vi "shag_start — 10.vi"() -> ()   [LabVIEW 2016]
uses:
  <vilib>/Instr/_visa.llb/VISA Configure Serial Port (Instr).vi
panel:
  out "положение в мин 4":i32
  out "text4":string
  out "4":i32
  out "3":i32
  out "положение в мин 3":i32
  out "text3":string
  out "text":string
  out "2":i32
  out "1":i32
  out "text2":string
  out "положение в мин 2":i32
  out "положение в мин 1":i32
  in  "all":T1(tab)
  out "положение шд 2":i32(knob) scale=-10.0..190.0
  out "текущее положение 2":string
  out "положение в минутах 2":string
  in  "Минуты 2":i32 min=-600 max=11400
  in  "Stop двигатель 2":bool
  in  "Вращение по градусам +  2":bool
  in  "Вращение по градусам -  2":bool
  in  "Вернуться в нулевое положение 2":bool
  in  "Задать текущее положение нулевым 2":bool
  in  "Установка минут 2":bool
  in  "Блокировать трубку №2":bool
  out "положение шд":i32(knob) scale=-10.0..190.0
  out "текущее положение":string
  out "положение в минутах 1":string
  in  "Минуты":i32 min=-600 max=11400
  in  "Stop двигатель":bool
  in  "Вращение по градусам +":bool
  in  "Вращение по градусам -":bool
  in  "Вернуться в нулевое положение":bool
  in  "Задать текущее положение нулевым":bool
  in  "Установка минут":bool
  in  "Блокировать зеркало №1":bool
  in  "stop":bool
  out "положение шд 3":i32(knob) scale=-10.0..190.0
  out "текущее положение 3":string
  out "положение в минутах 3":string
  in  "Минуты 3":i32 min=-600 max=11400
  in  "Stop двигатель 3":bool
  in  "Вращение по градусам +  3":bool
  in  "Вращение по градусам -  3":bool
  in  "Вернуться в нулевое положение 3":bool
  in  "Задать текущее положение нулевым 3":bool
  in  "Установка минут 3":bool
  in  "Блокировать стол №3":bool caption="Блокировать трубку №2"
  out "положение шд 4":i32(knob) scale=-10.0..190.0
  out "текущее положение 4":string
  out "положение в минутах 4":string
  in  "Минуты 4":i32 min=-600 max=11400
  in  "Stop двигатель 4":bool
  in  "Вращение по градусам +  4":bool
  in  "Вращение по градусам -  4":bool
  in  "Вернуться в нулевое положение 4":bool
  in  "Задать текущее положение нулевым 4":bool
  in  "Установка минут 4":bool
  in  "Блокировать стол №3 2":bool caption="Блокировать трубку №2"
  in  "Выберете COM порт":refnum<visa-resource-name>="COM1"
  in  "Скорость обмена данными":u32(ring)=19200 items=["9600"=9600, "19200"=19200, "38400"=38400, "57600"=57600]
  in  "Число бит на символ":u16=8 min=5 max=8 step=1
  in  "Контроль чётности":enum16{"None", "Odd", "Even", "Mark", "Space"}(ring)
  in  "Стоповый бит":u16(ring)=10 items=["1.0"=10, "1.5"=15, "2.0"=20]
  in  "Контроль переполнения":u16(ring) items=["None"=0, "XON/XOFF"=1, "RTS/CTS"=2, "DTR/DSR"=4]
  # "1 - адресс 1 двигателя\n2 - адресс 2 двигателя\n$0MV\\01+   - запуск всех двигателей в положительном направлении \n$0MS\\00   - остановка всех двигателей\n$0MJ\\04+\\00\\00\\01   - 1 шаг всех двигателей\n$0SS\\01\\10   - скорость 10 для всех двигателей"
  # "Ренгеновская трубка №2"
  # "Положение:"
  # "Зеркало №1"
  # "Положение:"
  # "Поворотный стол №3"
  # "Положение:"
  # "Счётчик №4"
  # "Положение:"
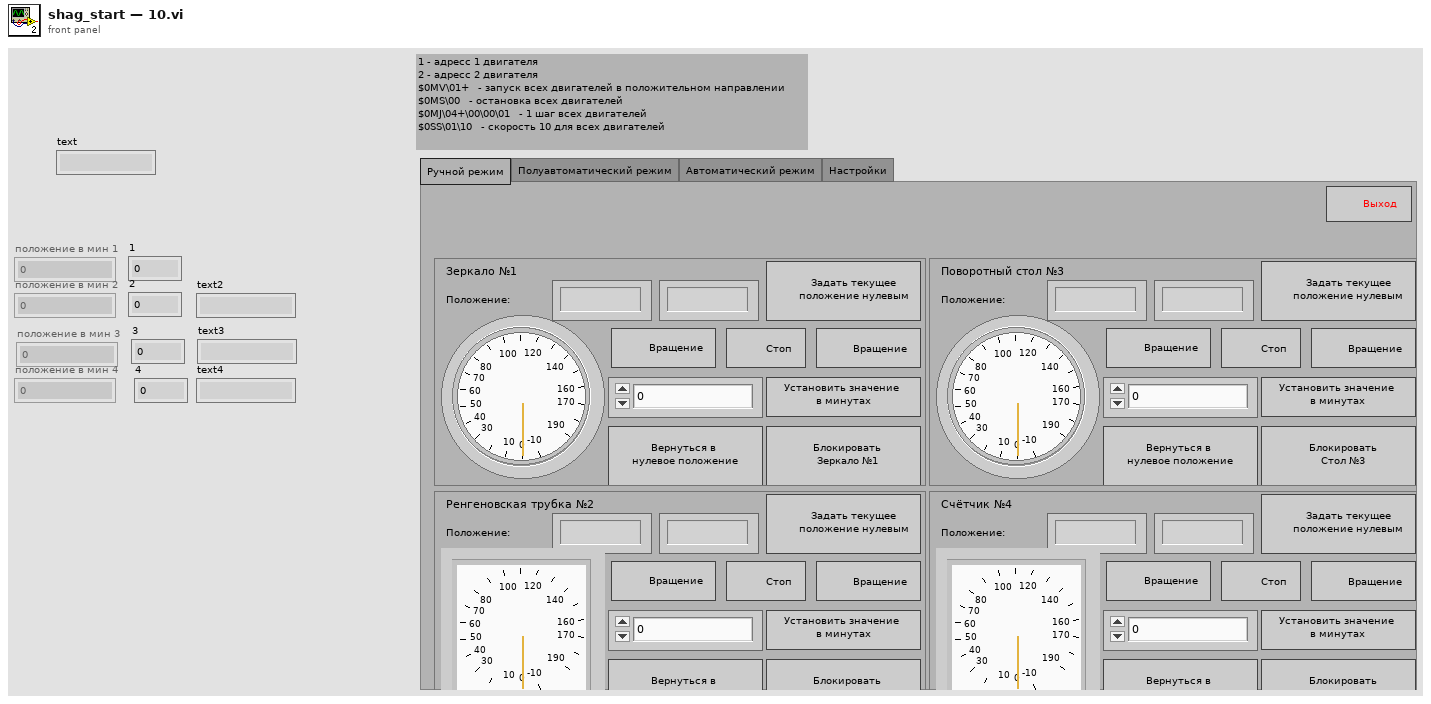
[diagram p1: front panel]
types:
  T1 = enum32{"Ручной режим", "Полуавтоматический режим", "Автоматический режим", "Настройки"}
  T2 = enum16{"open", "replace", "create", "open or create", "replace or create", "replace or create with confirmation"}
  T3 = enum8{"Enabled", "Disabled", "Disabled and Grayed Out"}
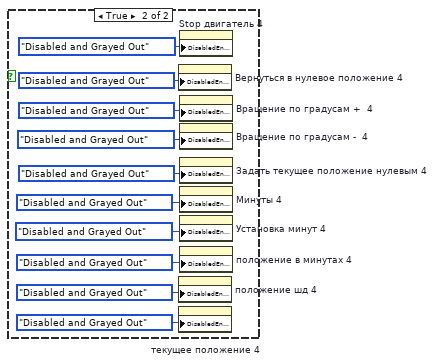
[diagram p2: hidden frame]
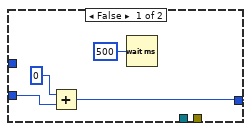
[diagram p4: hidden frame]
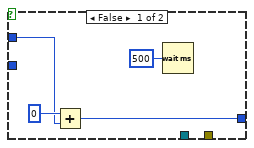
[diagram p5: hidden frame]
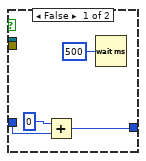
[diagram p7: hidden frame]
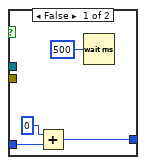
[diagram p8: hidden frame]
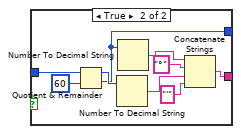
[diagram p9: hidden frame]
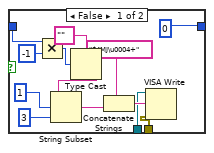
[diagram p11: hidden frame]
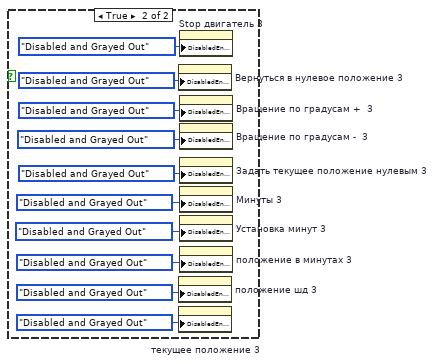
[diagram p13: hidden frame]
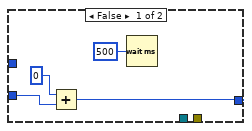
[diagram p15: hidden frame]
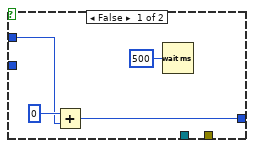
[diagram p16: hidden frame]
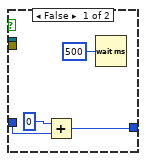
[diagram p18: hidden frame]
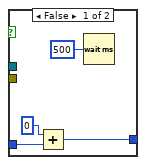
[diagram p19: hidden frame]
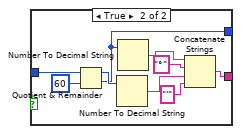
[diagram p20: hidden frame]
diagram:
  n1 = call-poly "VISA Configure Serial Port"("VISA resource name"="Выберете COM порт", "baud rate (9600)"="Скорость обмена данными", "data bits (8)"="Число бит на символ", "parity (0:none)"="Контроль чётности", "stop bits (10: 1 bit)"="Стоповый бит", "flow control (0:none)"="Контроль переполнения") -> ("VISA resource name out"=w32:refnum<visa-resource-name>, "error out"=w31:errorcluster)  [unwired: 8 in]
  n2 = Boolean To (0,1)(Boolean=FALSE ("DTR Write")) -> (0, 1=w33:i16)
  n3 = Boolean To (0,1)(Boolean=FALSE ("DTR Write")) -> (0, 1=w34:i16)
  n4 = property class="Instr"(reference=w32, error in=w31, "Serial Settings:Modem Line Settings:Line DTR State"=w33, "Serial Settings:Modem Line Settings:Line RTS State"=w34) -> (reference out=w30:refnum<visa-resource-name>, error out=w29:errorcluster)
  n5 = flat-sequence {
    tunnel: w30 -> [w63]
    tunnel: w29 -> [w62]
    tunnel: [w63] -> w28
    tunnel: [w62] -> w27
    tunnel: [w58] -> w18
    tunnel: [w66] -> w17
    tunnel: w28 -> [w66]
    tunnel: w27 -> [w65]
    tunnel: [w65] -> w15
    tunnel: [w66] -> w13
    tunnel: [w65] -> w11
    tunnel: w18 -> [w67]
    tunnel: [w65] -> w6
    tunnel: [w66] -> w5
    tunnel: [w66] -> w3
    tunnel: [w65] -> w1
    tunnel: w17 -> [w80]
    tunnel: [w80] -> w16
    tunnel: w15 -> [w79]
    tunnel: [w79] -> w14
    tunnel: w13 -> [w72]
    tunnel: [w72] -> w12
    tunnel: w11 -> [w74]
    tunnel: [w74] -> w10
    tunnel: [w75] -> w9
    tunnel: [w73] -> w8
    tunnel: [w71] -> w7
    tunnel: w6 -> [w73]
    tunnel: w5 -> [w71]
    tunnel: [w70] -> w4
    tunnel: w3 -> [w70]
    tunnel: [w69] -> w2
    tunnel: w1 -> [w69]
    tunnel: w16 -> [w90]
    tunnel: w14 -> [w89]
    tunnel: w12 -> [w85]
    tunnel: w10 -> [w88]
    tunnel: w9 -> [w87]
    tunnel: w8 -> [w84]
    tunnel: w7 -> [w83]
    tunnel: w4 -> [w82]
    tunnel: w2 -> [w81]
    frame #0 {
      n6 = VISA Write(VISA resource name=w63, write buffer="$0SS\u0001\u0010", error in (no error)=w62) -> ()  [unwired: 3 out]
      n7 = Open/Create/Replace File(file path (use dialog)=path "C:/Users/User/Desktop/shagovi_dvigatel/test_text_file", operation (0:open)=T2."open", access (0:read/write)=enum16{"read/write", "read-only", "write-only"}."read-only") -> (refnum out=w57:refnum<file>)  [unwired: 3 in, 2 out]
      n8 = Read from Text File(file (use dialog)=w57) -> (refnum out=w58:refnum<file>, text=w44:string)  [unwired: 3 in, 2 out]
      "text" <- w44
      n9 = Spreadsheet String To Array(delimiter (Tab)=" ", format string="%5f", spreadsheet string=w44) -> (array=w54:dbl[][])  [unwired: 1 in]
      n10 = Index Array(array=w54, index (row)=0 ("index")) -> (element=w52:dbl[])  [unwired: 1 in]
      n11 = Decimate 1D Array(w52) -> (w49:dbl[], w40:dbl[], w39:dbl[], w35:dbl[])
      n12 = Index Array(array=w35, index=0) -> (element=w37:dbl)
      n13 = Index Array(array=w39, index=0) -> (element=w42:dbl)
      n14 = Index Array(array=w40, index=0) -> (element=w48:dbl)
      n15 = To Long Integer(number=w37) -> (32bit integer=→"4":i32)
      n16 = To Long Integer(number=w42) -> (32bit integer=→"3":i32)
      n17 = Index Array(array=w49, index=0) -> (element=w47:dbl)
      n18 = To Long Integer(number=w48) -> (32bit integer=→"2":i32)
      n19 = To Long Integer(number=w47) -> (32bit integer=→"1":i32)
    }
    frame #1 {
      n20 = Close File(refnum=w67) -> ()  [unwired: 1 in, 2 out]
      n21 = Wait (ms)(milliseconds to wait=u32 500) -> ()  [unwired: 1 out]
    }
    frame #2 {
      n22 = Open/Create/Replace File(file path (use dialog)=path "C:/Users/User/Desktop/shagovi_dvigatel/test_text_file", operation (0:open)=T2."replace or create", access (0:read/write)=enum16{"read/write", "read-only", "write-only"}."write-only") -> (refnum out=w75:refnum<file>)  [unwired: 3 in, 2 out]
    }
    frame #3 {
      n23 = while {
        tunnel: w90 -> [w197]
        tunnel: w89 -> [w196]
        shift-right: [w192] -> _
        shift-left: _ -> [w201]
        shift-right: [w193] -> _
        shift-left: _ -> [w200]
        shift-right: [w194] -> _
        shift-left: _ -> [w199]
        shift-right: [w195] -> _
        shift-left: _ -> [w198]
        tunnel: w88 -> [w166]
        shift-right: [w188] -> w86
        shift-left: w87 -> [w189]
        tunnel: w85 -> [w165]
        shift-right: [w161] -> _
        shift-left: _ -> [w162]
        shift-right: [w159] -> _
        shift-left: _ -> [w160]
        shift-right: [w157] -> _
        shift-left: _ -> [w158]
        shift-right: [w155] -> _
        shift-left: _ -> [w156]
        tunnel: w84 -> [w133]
        tunnel: w83 -> [w132]
        shift-right: [w129] -> _
        shift-left: _ -> [w130]
        shift-right: [w127] -> _
        shift-left: _ -> [w128]
        shift-right: [w125] -> _
        shift-left: _ -> [w126]
        shift-right: [w123] -> _
        shift-left: _ -> [w124]
        tunnel: w82 -> [w101]
        tunnel: w81 -> [w100]
        shift-right: [w97] -> _
        shift-left: _ -> [w98]
        shift-right: [w95] -> _
        shift-left: _ -> [w96]
        shift-right: [w93] -> _
        shift-left: _ -> [w94]
        shift-right: [w91] -> _
        shift-left: _ -> [w92]
        stop <- "stop" stop-if-true
        # "Управление вращением"
        # "Управление вращением"
        n24 = flat-sequence {
          tunnel: w133 -> [w522]
          tunnel: w132 -> [w523]
          tunnel: [w523] -> w154
          tunnel: [w522] -> w153
          tunnel: ["Вращение по градусам +  3"] -> w152
          tunnel: ["Вращение по градусам -  3"] -> w151
          tunnel: ["Вернуться в нулевое положение 3"] -> w150
          tunnel: ["Задать текущее положение нулевым 3"] -> w149
          tunnel: ["Установка минут 3"] -> w148
          tunnel: w154 -> [w547]
          tunnel: w153 -> [w531]
          tunnel: [w570] -> w147
          tunnel: w130 -> [w567]
          tunnel: w128 -> [w569]
          tunnel: [w568] -> w146
          tunnel: w126 -> [w566]
          tunnel: w124 -> [w565]
          tunnel: w152 -> [w551]
          tunnel: w151 -> [w550]
          tunnel: [w564] -> w145
          tunnel: [w563] -> w144
          tunnel: [w548] -> w143
          tunnel: w150 -> [w548]
          tunnel: [w531] -> w142
          tunnel: [w547] -> w141
          tunnel: [w546] -> w140
          tunnel: w149 -> [w546]
          tunnel: w148 -> [w540]
          tunnel: [w529] -> w139
          tunnel: w147 -> [w654]
          tunnel: w146 -> [w655]
          tunnel: [w672] -> w138
          tunnel: [w670] -> w137
          tunnel: w145 -> [w656]
          tunnel: w144 -> [w657]
          tunnel: [w661] -> w136
          tunnel: [w668] -> w135
          tunnel: w143 -> [w664]
          tunnel: w142 -> [w660]
          tunnel: w141 -> [w659]
          tunnel: w140 -> [w658]
          tunnel: [w658] -> w134
          tunnel: w139 -> [w644]
          tunnel: [w752] -> w129
          tunnel: [w749] -> w127
          tunnel: w138 -> [w751]
          tunnel: w137 -> [w750]
          tunnel: [w748] -> w125
          tunnel: [w747] -> w123
          tunnel: w136 -> [w746]
          tunnel: w135 -> [w745]
          tunnel: w134 -> [w744]
          frame #0 {
            n25 = Wait Until Next ms Multiple(millisecond multiple=u32 300) -> ()  [unwired: 1 out]
          }
          frame #1 {
            # "Остановка двигателя"
            n26 = Greater?(x="Минуты 3", y=0) -> (0:w538:bool)
            n27 = case shown="True" "Stop двигатель 3" {
              tunnel: w547 -> [_ w618]
              tunnel: w531 -> [_ w617]
              frame False {
              }
              frame True {
                n28 = Wait (ms)(milliseconds to wait=u32 500) -> ()  [unwired: 1 out]
                n29 = VISA Write(VISA resource name=w618, write buffer="$3MS\u0001", error in (no error)=w617) -> ()  [unwired: 3 out]
              }
            }
            n30 = Not Equal?(x="Минуты 3", y=0) -> (x != y?=w537:bool)
            n31 = local read "положение в мин 3"() -> (w530:i32)
            n32 = Add(x="Минуты 3", y=w530) -> (x+y=w561:i32)
            n33 = Add(x="Минуты 3", y=w530) -> (x+y=w533:i32)
            n34 = Not Equal?(x="Минуты 3", y=0) -> (x != y?=w535:bool)
            n35 = Add(x=w530, y=60) -> (x+y=w556:i32)
            n36 = Subtract(x=w530, y=60) -> (x-y=w543:i32)
            n37 = Not(x=w538) -> (.not. x?=w539:bool)
            n38 = Greater Or Equal?(x=w533, y=-600) -> (x >= y?=w534:bool)
            n39 = Less Or Equal?(x=w561, y=11400) -> (x <= y?=w536:bool)
            n40 = Less Or Equal?(x=w556, y=11390) -> (x <= y?=w553:bool)
            n41 = Greater Or Equal?(x=w543, y=-590) -> (x >= y?=w544:bool)
            n42 = Compound Arithmetic op=AND(w539, w535, w534) -> (w557:bool)
            n43 = And(x=w551, y=w553) -> (x .and. y?=w552:bool)
            n44 = And(x=w550, y=w544) -> (x .and. y?=w549:bool)
            n45 = Compound Arithmetic op=AND(w538, w537, w536) -> (w559:bool)
            n46 = case shown="True" w540 {
              tunnel: [w573 w582] -> w570
              tunnel: w569 -> [w572 w581]
              tunnel: [w572 w580] -> w568
              tunnel: w567 -> [w573 w579]
              tunnel: w559 -> [_ w578]
              tunnel: w557 -> [_ w577]
              tunnel: w531 -> [_ w576]
              tunnel: w547 -> [_ w575]
              tunnel: "Минуты 3" -> [_ w574]
              frame False {
              }
              frame True {
                n47 = case shown="True" w578 {
                  tunnel: [w603 w609] -> w582
                  tunnel: w579 -> [w602 w608]
                  tunnel: w576 -> [_ w607]
                  tunnel: w575 -> [_ w606]
                  tunnel: w574 -> [_ w605]
                  frame False {
                    n48 = Add(x=0, y=w602) -> (x+y=w603:i32)
                    n49 = Wait (ms)(milliseconds to wait=u32 500) -> ()  [unwired: 1 out]
                  }
                  frame True {
                    n50 = Type Cast(type="", x=w605) -> (*(type *) &x=w612:string)
                    n51 = Add(x=w605, y=w608) -> (x+y=w609:i32)
                    n52 = String Subset(string=w612, offset (0)=1, length (rest)=3 ("length (rest)")) -> (substring=w611:string)
                    n53 = Concatenate Strings("$3MJ\u0004+" ("write buffer"), w611) -> (w615:string)
                    n54 = VISA Write(VISA resource name=w606, write buffer=w615, error in (no error)=w607) -> ()  [unwired: 3 out]
                  }
                }
                n55 = case shown="True" w577 {
                  tunnel: [w585 w591] -> w580
                  tunnel: w581 -> [w584 w590]
                  tunnel: w575 -> [_ w593]
                  tunnel: w576 -> [_ w592]
                  tunnel: w574 -> [_ w587]
                  frame False {
                    n56 = Add(x=0, y=w584) -> (x+y=w585:i32)
                    n57 = Wait (ms)(milliseconds to wait=u32 500) -> ()  [unwired: 1 out]
                  }
                  frame True {
                    n58 = Multiply(x=w587, y=-1) -> (x*y=w589:i32)
                    n59 = Type Cast(type="", x=w589) -> (*(type *) &x=w596:string)
                    n60 = Add(x=w590, y=w587) -> (x+y=w591:i32)
                    n61 = String Subset(string=w596, offset (0)=1, length (rest)=3 ("length (rest)")) -> (substring=w595:string)
                    n62 = Concatenate Strings("$3MJ\u0004-" ("write buffer"), w595) -> (w599:string)
                    n63 = VISA Write(VISA resource name=w593, write buffer=w599, error in (no error)=w592) -> ()  [unwired: 3 out]
                  }
                }
              }
            }
            n64 = case shown="True" w552 {
              tunnel: [w633 w640] -> w564
              tunnel: w566 -> [w632 w635]
              tunnel: w547 -> [_ w636]
              tunnel: w531 -> [_ w637]
              frame False {
                n65 = Add(x=0, y=w632) -> (x+y=w633:i32)
                n66 = Wait (ms)(milliseconds to wait=u32 500) -> ()  [unwired: 1 out]
              }
              frame True {
                n67 = VISA Write(VISA resource name=w636, write buffer="$3MJ\u0004+\u0000\u0000<", error in (no error)=w637) -> ()  [unwired: 3 out]
                n68 = Add(x=60, y=w635) -> (x+y=w640:i32)
              }
            }
            n69 = case shown="True" w549 {
              tunnel: [w623 w626] -> w563
              tunnel: w565 -> [w622 w625]
              tunnel: w547 -> [_ w629]
              tunnel: w531 -> [_ w628]
              frame False {
                n70 = Add(x=0, y=w622) -> (x+y=w623:i32)
                n71 = Wait (ms)(milliseconds to wait=u32 500) -> ()  [unwired: 1 out]
              }
              frame True {
                n72 = Subtract(x=w625, y=60 ("x")) -> (x-y=w626:i32)
                n73 = VISA Write(VISA resource name=w629, write buffer="$3MJ\u0004-\u0000\u0000<", error in (no error)=w628) -> ()  [unwired: 3 out]
              }
            }
            n74 = for {
              N: 1 -> [_]
              tunnel: [w571] -> w527 mode=indexing
              n75 = local read "3"() -> (w571:i32)
            }
            n76 = Index Array(array=w527, index=0) -> (element=w529:i32)
          }
          frame #2 {
            # "Нулевое положение"
            n77 = Add(x=w656, y=w657) -> (x+y=w665:i32)
            n78 = Add(x=w654, y=w655) -> (x+y=w669:i32)
            n79 = Add(x=w669, y=w665) -> (x+y=w650:i32)
            n80 = Add(x=w650, y=w644) -> (x+y=w649:i32)
            n81 = Not Equal?(x=w649, y=0 ("x")) -> (x != y?=w662:bool)
            n82 = And(x=w662, y=w664) -> (x .and. y?=w671:bool)
            n83 = case shown="True" w671 {
              tunnel: [w696 w719] -> w646
              tunnel: w654 -> [w700 w716]
              tunnel: [w700 w715] -> w672
              tunnel: [w699 w714] -> w670
              tunnel: w649 -> [w696 w708]
              tunnel: [w697 w710] -> w668
              tunnel: [w698 w707] -> w661
              tunnel: w655 -> [w699 w706]
              tunnel: w660 -> [_ w705]
              tunnel: w659 -> [_ w704]
              tunnel: w656 -> [w698 w703]
              tunnel: w657 -> [w697 w702]
              frame False {
              }
              frame True {
                n84 = Greater?(x=w708, y=0) -> (0:w709:bool)
                n85 = Multiply(x=w702, y=0) -> (x*y=w710:i32)
                n86 = Multiply(x=w706, y=0) -> (x*y=w714:i32)
                n87 = case shown="False" w709 {
                  tunnel: w708 -> [w724 w737]
                  tunnel: [0 0] -> w719
                  tunnel: w704 -> [w721 w734]
                  tunnel: w705 -> [w720 w733]
                  frame False {
                    n88 = Multiply(x=w724, y=-1) -> (x*y=w722:i32)
                    n89 = Type Cast(type="", x=w722) -> (*(type *) &x=w728:string)
                    n90 = String Subset(string=w728, offset (0)=1, length (rest)=3 ("length (rest)")) -> (substring=w727:string)
                    n91 = Concatenate Strings("$3MJ\u0004+" ("write buffer"), w727) -> (w731:string)
                    n92 = VISA Write(VISA resource name=w721, write buffer=w731, error in (no error)=w720) -> ()  [unwired: 3 out]
                  }
                  frame True {
                    n93 = Type Cast(type="", x=w737) -> (*(type *) &x=w740:string)
                    n94 = String Subset(string=w740, offset (0)=1, length (rest)=3 ("length (rest)")) -> (substring=w739:string)
                    n95 = Concatenate Strings("$3MJ\u0004-" ("write buffer"), w739) -> (w735:string)
                    n96 = VISA Write(VISA resource name=w734, write buffer=w735, error in (no error)=w733) -> ()  [unwired: 3 out]
                  }
                }
                n97 = local write "3"(0 ("3")) -> ()
                n98 = Multiply(x=w703, y=0) -> (x*y=w707:i32)
                n99 = Multiply(x=w716, y=0) -> (x*y=w715:i32)
              }
            }
            "положение в мин 3" <- w646
            n100 = Greater?(x=w646, y=0) -> (0:w667:bool)
            n101 = Number To Decimal String(number=w646, width (-)=i16 1) -> (decimal integer string=w652:string)
            n102 = case shown="False" w667 {
              tunnel: w646 -> [w679 w695]
              tunnel: [w683 w689] -> w643
              tunnel: [w673 w687] -> w641
              frame False {
                n103 = Multiply(x=-1, y=w679) -> (x*y=w678:i32)
                n104 = Quotient & Remainder(x=w678, y=60) -> (x-y*floor(x/y)=w682:i32, floor(x/y)=w674:i32)
                n105 = Multiply(x=-1, y=w674) -> (x*y=w673:i32)
                n106 = Number To Decimal String(number=w674) -> (decimal integer string=w680:string)  [unwired: 1 in]
                n107 = Number To Decimal String(number=w682) -> (decimal integer string=w681:string)  [unwired: 1 in]
                n108 = Concatenate Strings("-" ("string"), w680, "°" ("string"), w681, "'" ("string")) -> (w683:string)
              }
              frame True {
                n109 = Quotient & Remainder(x=w695, y=60) -> (x-y*floor(x/y)=w688:i32, floor(x/y)=w687:i32)
                n110 = Number To Decimal String(number=w688) -> (decimal integer string=w690:string)  [unwired: 1 in]
                n111 = Number To Decimal String(number=w687) -> (decimal integer string=w691:string)  [unwired: 1 in]
                n112 = Concatenate Strings(w691, "°" ("string"), w690, "'" ("string")) -> (w689:string)
              }
            }
            "текущее положение 3" <- w643
            "положение шд 3" <- w641
            n113 = Concatenate Strings(w652, "'" ("string")) -> (→"положение в минутах 3":string)
            n114 = Format Into String(w646) -> (resulting string=w647:string)  [unwired: 3 in, 1 out]
            n115 = call <vilib>:"Space Constant.vi"() -> ("String"=w645:string)
            n116 = Concatenate Strings(w645, w647) -> (→"text3":string)
          }
          frame #3 {
            # "Задача нуля"
            n117 = case shown="True" w744 {
              tunnel: [w756 w768] -> w752
              tunnel: w751 -> [w756 w769]
              tunnel: w750 -> [w755 w765]
              tunnel: [w755 w764] -> w749
              tunnel: [w754 w761] -> w748
              tunnel: [w753 w760] -> w747
              tunnel: w746 -> [w754 w759]
              tunnel: w745 -> [w753 w758]
              frame False {
              }
              frame True {
                n118 = Multiply(x=w765, y=0) -> (x*y=w764:i32)
                n119 = Multiply(x=w769, y=0) -> (x*y=w768:i32)
                n120 = Multiply(x=w758, y=0) -> (x*y=w760:i32)
                n121 = Multiply(x=w759, y=0) -> (x*y=w761:i32)
                n122 = local write "3"(0 ("3")) -> ()
              }
            }
          }
        }
        n123 = flat-sequence {
          tunnel: w196 -> [w1070]
          tunnel: w197 -> [w1071]
          tunnel: [w1071] -> w221
          tunnel: [w1070] -> w220
          tunnel: ["Вращение по градусам +"] -> w219
          tunnel: ["Вращение по градусам -"] -> w218
          tunnel: ["Вернуться в нулевое положение"] -> w217
          tunnel: ["Задать текущее положение нулевым"] -> w216
          tunnel: ["Установка минут"] -> w215
          tunnel: w221 -> [w1095]
          tunnel: w220 -> [w1077]
          tunnel: [w1118] -> w214
          tunnel: w201 -> [w1115]
          tunnel: w200 -> [w1117]
          tunnel: [w1116] -> w213
          tunnel: w199 -> [w1114]
          tunnel: w198 -> [w1113]
          tunnel: w219 -> [w1099]
          tunnel: w218 -> [w1098]
          tunnel: [w1112] -> w212
          tunnel: [w1111] -> w211
          tunnel: [w1096] -> w210
          tunnel: w217 -> [w1096]
          tunnel: [w1077] -> w209
          tunnel: [w1095] -> w208
          tunnel: [w1094] -> w207
          tunnel: w216 -> [w1094]
          tunnel: w215 -> [w1088]
          tunnel: [w1075] -> w190
          tunnel: w214 -> [w1200]
          tunnel: w213 -> [w1201]
          tunnel: [w1220] -> w206
          tunnel: [w1218] -> w205
          tunnel: w212 -> [w1202]
          tunnel: w211 -> [w1203]
          tunnel: [w1209] -> w204
          tunnel: [w1216] -> w203
          tunnel: w210 -> [w1212]
          tunnel: w209 -> [w1208]
          tunnel: w208 -> [w1207]
          tunnel: w207 -> [w1205]
          tunnel: [w1205] -> w202
          tunnel: [w1194] -> _
          tunnel: "stop" -> [w1197]
          tunnel: w189 -> [w1194]
          tunnel: w190 -> [w1189]
          tunnel: [w1190] -> w188
          tunnel: [w1309] -> w192
          tunnel: [w1306] -> w193
          tunnel: w206 -> [w1308]
          tunnel: w205 -> [w1307]
          tunnel: [w1305] -> w194
          tunnel: [w1304] -> w195
          tunnel: w204 -> [w1303]
          tunnel: w203 -> [w1302]
          tunnel: w202 -> [w1301]
          frame #0 {
            n124 = Wait Until Next ms Multiple(millisecond multiple=u32 300) -> ()  [unwired: 1 out]
          }
          frame #1 {
            # "Остановка двигателя"
            n125 = Greater?(x="Минуты", y=0) -> (0:w1086:bool)
            n126 = case shown="True" "Stop двигатель" {
              tunnel: w1095 -> [_ w1166]
              tunnel: w1077 -> [_ w1165]
              frame False {
              }
              frame True {
                n127 = Wait (ms)(milliseconds to wait=u32 500) -> ()  [unwired: 1 out]
                n128 = VISA Write(VISA resource name=w1166, write buffer="$1MS\u0001", error in (no error)=w1165) -> ()  [unwired: 3 out]
              }
            }
            n129 = Not Equal?(x="Минуты", y=0) -> (x != y?=w1085:bool)
            n130 = local read "положение в мин 1"() -> (w1076:i32)
            n131 = Add(x="Минуты", y=w1076) -> (x+y=w1109:i32)
            n132 = Add(x="Минуты", y=w1076) -> (x+y=w1080:i32)
            n133 = Not Equal?(x="Минуты", y=0) -> (x != y?=w1083:bool)
            n134 = Add(x=w1076, y=60) -> (x+y=w1104:i32)
            n135 = Subtract(x=w1076, y=60) -> (x-y=w1091:i32)
            n136 = Not(x=w1086) -> (.not. x?=w1087:bool)
            n137 = Greater Or Equal?(x=w1080, y=-600) -> (x >= y?=w1081:bool)
            n138 = Less Or Equal?(x=w1109, y=11400) -> (x <= y?=w1084:bool)
            n139 = Less Or Equal?(x=w1104, y=11390) -> (x <= y?=w1101:bool)
            n140 = Greater Or Equal?(x=w1091, y=-590) -> (x >= y?=w1092:bool)
            n141 = Compound Arithmetic op=AND(w1087, w1083, w1081) -> (w1105:bool)
            n142 = And(x=w1099, y=w1101) -> (x .and. y?=w1100:bool)
            n143 = And(x=w1098, y=w1092) -> (x .and. y?=w1097:bool)
            n144 = Compound Arithmetic op=AND(w1086, w1085, w1084) -> (w1107:bool)
            n145 = case shown="True" w1088 {
              tunnel: [w1121 w1130] -> w1118
              tunnel: w1117 -> [w1120 w1129]
              tunnel: [w1120 w1128] -> w1116
              tunnel: w1115 -> [w1121 w1127]
              tunnel: w1107 -> [_ w1126]
              tunnel: w1105 -> [_ w1125]
              tunnel: w1077 -> [_ w1124]
              tunnel: w1095 -> [_ w1123]
              tunnel: "Минуты" -> [_ w1122]
              frame False {
              }
              frame True {
                n146 = case shown="True" w1126 {
                  tunnel: [w1151 w1157] -> w1130
                  tunnel: w1127 -> [w1150 w1156]
                  tunnel: w1124 -> [_ w1155]
                  tunnel: w1123 -> [_ w1154]
                  tunnel: w1122 -> [_ w1153]
                  frame False {
                    n147 = Add(x=0, y=w1150) -> (x+y=w1151:i32)
                    n148 = Wait (ms)(milliseconds to wait=u32 500) -> ()  [unwired: 1 out]
                  }
                  frame True {
                    n149 = Type Cast(type="", x=w1153) -> (*(type *) &x=w1160:string)
                    n150 = Add(x=w1153, y=w1156) -> (x+y=w1157:i32)
                    n151 = String Subset(string=w1160, offset (0)=1, length (rest)=3 ("length (rest)")) -> (substring=w1159:string)
                    n152 = Concatenate Strings("$1MJ\u0004+" ("write buffer"), w1159) -> (w1163:string)
                    n153 = VISA Write(VISA resource name=w1154, write buffer=w1163, error in (no error)=w1155) -> ()  [unwired: 3 out]
                  }
                }
                n154 = case shown="True" w1125 {
                  tunnel: [w1133 w1139] -> w1128
                  tunnel: w1129 -> [w1132 w1138]
                  tunnel: w1123 -> [_ w1141]
                  tunnel: w1124 -> [_ w1140]
                  tunnel: w1122 -> [_ w1135]
                  frame False {
                    n155 = Add(x=0, y=w1132) -> (x+y=w1133:i32)
                    n156 = Wait (ms)(milliseconds to wait=u32 500) -> ()  [unwired: 1 out]
                  }
                  frame True {
                    n157 = Multiply(x=w1135, y=-1) -> (x*y=w1137:i32)
                    n158 = Type Cast(type="", x=w1137) -> (*(type *) &x=w1144:string)
                    n159 = Add(x=w1138, y=w1135) -> (x+y=w1139:i32)
                    n160 = String Subset(string=w1144, offset (0)=1, length (rest)=3 ("length (rest)")) -> (substring=w1143:string)
                    n161 = Concatenate Strings("$1MJ\u0004-" ("write buffer"), w1143) -> (w1147:string)
                    n162 = VISA Write(VISA resource name=w1141, write buffer=w1147, error in (no error)=w1140) -> ()  [unwired: 3 out]
                  }
                }
              }
            }
            n163 = case shown="True" w1100 {
              tunnel: [w1181 w1188] -> w1112
              tunnel: w1114 -> [w1180 w1183]
              tunnel: w1095 -> [_ w1184]
              tunnel: w1077 -> [_ w1185]
              frame False {
                n164 = Add(x=0, y=w1180) -> (x+y=w1181:i32)
                n165 = Wait (ms)(milliseconds to wait=u32 500) -> ()  [unwired: 1 out]
              }
              frame True {
                n166 = VISA Write(VISA resource name=w1184, write buffer="$1MJ\u0004+\u0000\u0000<", error in (no error)=w1185) -> ()  [unwired: 3 out]
                n167 = Add(x=60, y=w1183) -> (x+y=w1188:i32)
              }
            }
            n168 = case shown="True" w1097 {
              tunnel: [w1171 w1174] -> w1111
              tunnel: w1113 -> [w1170 w1173]
              tunnel: w1095 -> [_ w1177]
              tunnel: w1077 -> [_ w1176]
              frame False {
                n169 = Add(x=0, y=w1170) -> (x+y=w1171:i32)
                n170 = Wait (ms)(milliseconds to wait=u32 500) -> ()  [unwired: 1 out]
              }
              frame True {
                n171 = Subtract(x=w1173, y=60 ("x")) -> (x-y=w1174:i32)
                n172 = VISA Write(VISA resource name=w1177, write buffer="$1MJ\u0004-\u0000\u0000<", error in (no error)=w1176) -> ()  [unwired: 3 out]
              }
            }
            n173 = for {
              N: 1 -> [_]
              tunnel: [w1119] -> w1073 mode=indexing
              n174 = local read "1"() -> (w1119:i32)
            }
            n175 = Index Array(array=w1073, index=0) -> (element=w1075:i32)
          }
          frame #2 {
            # "Нулевое положение"
            n176 = Add(x=w1202, y=w1203) -> (x+y=w1213:i32)
            n177 = Add(x=w1200, y=w1201) -> (x+y=w1217:i32)
            n178 = Add(x=w1217, y=w1213) -> (x+y=w1192:i32)
            n179 = Add(x=w1192, y=w1189) -> (x+y=w1191:i32)
            n180 = Not Equal?(x=w1191, y=0 ("x")) -> (x != y?=w1210:bool)
            n181 = And(x=w1210, y=w1212) -> (x .and. y?=w1219:bool)
            n182 = case shown="True" w1219 {
              tunnel: [w1253 w1276] -> w1193
              tunnel: w1200 -> [w1257 w1273]
              tunnel: [w1257 w1272] -> w1220
              tunnel: [w1256 w1271] -> w1218
              tunnel: w1191 -> [w1253 w1265]
              tunnel: [w1254 w1267] -> w1216
              tunnel: [w1255 w1264] -> w1209
              tunnel: w1201 -> [w1256 w1263]
              tunnel: w1208 -> [_ w1262]
              tunnel: w1207 -> [_ w1261]
              tunnel: w1202 -> [w1255 w1260]
              tunnel: w1203 -> [w1254 w1259]
              frame False {
              }
              frame True {
                n183 = Greater?(x=w1265, y=0) -> (0:w1266:bool)
                n184 = Multiply(x=w1259, y=0) -> (x*y=w1267:i32)
                n185 = Multiply(x=w1263, y=0) -> (x*y=w1271:i32)
                n186 = case shown="True" w1266 {
                  tunnel: w1265 -> [w1281 w1294]
                  tunnel: [0 0] -> w1276
                  tunnel: w1261 -> [w1278 w1291]
                  tunnel: w1262 -> [w1277 w1290]
                  frame False {
                    n187 = Multiply(x=w1281, y=-1) -> (x*y=w1279:i32)
                    n188 = Type Cast(type="", x=w1279) -> (*(type *) &x=w1285:string)
                    n189 = String Subset(string=w1285, offset (0)=1, length (rest)=3 ("length (rest)")) -> (substring=w1284:string)
                    n190 = Concatenate Strings("$1MJ\u0004+" ("write buffer"), w1284) -> (w1288:string)
                    n191 = VISA Write(VISA resource name=w1278, write buffer=w1288, error in (no error)=w1277) -> ()  [unwired: 3 out]
                  }
                  frame True {
                    n192 = Type Cast(type="", x=w1294) -> (*(type *) &x=w1297:string)
                    n193 = String Subset(string=w1297, offset (0)=1, length (rest)=3 ("length (rest)")) -> (substring=w1296:string)
                    n194 = Concatenate Strings("$1MJ\u0004-" ("write buffer"), w1296) -> (w1292:string)
                    n195 = VISA Write(VISA resource name=w1291, write buffer=w1292, error in (no error)=w1290) -> ()  [unwired: 3 out]
                  }
                }
                n196 = Multiply(x=w1260, y=0) -> (x*y=w1264:i32)
                n197 = Multiply(x=w1273, y=0) -> (x*y=w1272:i32)
                n198 = local write "1"(0 ("1")) -> ()
              }
            }
            "положение в мин 1" <- w1193
            n199 = Greater?(x=w1193, y=0) -> (0:w1215:bool)
            n200 = Number To Decimal String(number=w1193, width (-)=i16 1) -> (decimal integer string=w1196:string)
            n201 = case shown="True" w1197 {
              tunnel: w1194 -> [w1221 w1228]
              tunnel: w1193 -> [_ w1229]
              tunnel: [w1221 w1227] -> w1190
              frame False {
              }
              frame True {
                n202 = Format Into String(w1229) -> (resulting string=w1225:string)  [unwired: 3 in, 1 out]
                n203 = local read "text2"() -> (w1224:string)
                n204 = local read "text3"() -> (w1223:string)
                n205 = local read "text4"() -> (w1222:string)
                n206 = Concatenate Strings(w1225, w1224, w1223, w1222) -> (w1226:string)
                n207 = Write to Text File(file (use dialog)=w1228, text=w1226) -> (refnum out=w1227:refnum<file>)  [unwired: 2 in, 2 out]
              }
            }
            n208 = case shown="False" w1215 {
              tunnel: w1193 -> [w1236 w1252]
              tunnel: [w1240 w1246] -> w1206
              tunnel: [w1230 w1244] -> w1204
              frame False {
                n209 = Multiply(x=-1, y=w1236) -> (x*y=w1235:i32)
                n210 = Quotient & Remainder(x=w1235, y=60) -> (x-y*floor(x/y)=w1239:i32, floor(x/y)=w1231:i32)
                n211 = Multiply(x=-1, y=w1231) -> (x*y=w1230:i32)
                n212 = Number To Decimal String(number=w1231) -> (decimal integer string=w1237:string)  [unwired: 1 in]
                n213 = Number To Decimal String(number=w1239) -> (decimal integer string=w1238:string)  [unwired: 1 in]
                n214 = Concatenate Strings("-" ("string"), w1237, "°" ("string"), w1238, "'" ("string")) -> (w1240:string)
              }
              frame True {
                n215 = Quotient & Remainder(x=w1252, y=60) -> (x-y*floor(x/y)=w1245:i32, floor(x/y)=w1244:i32)
                n216 = Number To Decimal String(number=w1245) -> (decimal integer string=w1247:string)  [unwired: 1 in]
                n217 = Number To Decimal String(number=w1244) -> (decimal integer string=w1248:string)  [unwired: 1 in]
                n218 = Concatenate Strings(w1248, "°" ("string"), w1247, "'" ("string")) -> (w1246:string)
              }
            }
            "положение шд" <- w1204
            "текущее положение" <- w1206
            n219 = Concatenate Strings(w1196, "'" ("string")) -> (→"положение в минутах 1":string)
          }
          frame #3 {
            # "Задача нуля"
            n220 = case shown="True" w1301 {
              tunnel: [w1313 w1325] -> w1309
              tunnel: w1308 -> [w1313 w1326]
              tunnel: w1307 -> [w1312 w1322]
              tunnel: [w1312 w1321] -> w1306
              tunnel: [w1311 w1318] -> w1305
              tunnel: [w1310 w1317] -> w1304
              tunnel: w1303 -> [w1311 w1316]
              tunnel: w1302 -> [w1310 w1315]
              frame False {
              }
              frame True {
                n221 = Multiply(x=w1322, y=0) -> (x*y=w1321:i32)
                n222 = Multiply(x=w1326, y=0) -> (x*y=w1325:i32)
                n223 = local write "1"(0 ("1")) -> ()
                n224 = Multiply(x=w1315, y=0) -> (x*y=w1317:i32)
                n225 = Multiply(x=w1316, y=0) -> (x*y=w1318:i32)
              }
            }
          }
        }
        n226 = flat-sequence {
          tunnel: w166 -> [w796]
          tunnel: w165 -> [w797]
          tunnel: [w797] -> w187
          tunnel: [w796] -> w186
          tunnel: ["Вращение по градусам +  2"] -> w185
          tunnel: ["Вращение по градусам -  2"] -> w184
          tunnel: ["Вернуться в нулевое положение 2"] -> w183
          tunnel: ["Задать текущее положение нулевым 2"] -> w182
          tunnel: ["Установка минут 2"] -> w181
          tunnel: w187 -> [w821]
          tunnel: w186 -> [w805]
          tunnel: [w844] -> w180
          tunnel: w162 -> [w841]
          tunnel: w160 -> [w843]
          tunnel: [w842] -> w179
          tunnel: w158 -> [w840]
          tunnel: w156 -> [w839]
          tunnel: w185 -> [w825]
          tunnel: w184 -> [w824]
          tunnel: [w838] -> w178
          tunnel: [w837] -> w177
          tunnel: [w822] -> w176
          tunnel: w183 -> [w822]
          tunnel: [w805] -> w175
          tunnel: [w821] -> w174
          tunnel: [w820] -> w173
          tunnel: w182 -> [w820]
          tunnel: w181 -> [w814]
          tunnel: [w803] -> w172
          tunnel: w180 -> [w928]
          tunnel: w179 -> [w929]
          tunnel: [w946] -> w171
          tunnel: [w944] -> w170
          tunnel: w178 -> [w930]
          tunnel: w177 -> [w931]
          tunnel: [w935] -> w169
          tunnel: [w942] -> w168
          tunnel: w176 -> [w938]
          tunnel: w175 -> [w934]
          tunnel: w174 -> [w933]
          tunnel: w173 -> [w932]
          tunnel: [w932] -> w167
          tunnel: w172 -> [w915]
          tunnel: [w1026] -> w161
          tunnel: [w1023] -> w159
          tunnel: w171 -> [w1025]
          tunnel: w170 -> [w1024]
          tunnel: [w1022] -> w157
          tunnel: [w1021] -> w155
          tunnel: w169 -> [w1020]
          tunnel: w168 -> [w1019]
          tunnel: w167 -> [w1018]
          frame #0 {
            n227 = Wait Until Next ms Multiple(millisecond multiple=u32 300) -> ()  [unwired: 1 out]
          }
          frame #1 {
            # "Остановка двигателя"
            n228 = Greater?(x="Минуты 2", y=0) -> (0:w812:bool)
            n229 = case shown="True" "Stop двигатель 2" {
              tunnel: w821 -> [_ w892]
              tunnel: w805 -> [_ w891]
              frame False {
              }
              frame True {
                n230 = Wait (ms)(milliseconds to wait=u32 500) -> ()  [unwired: 1 out]
                n231 = VISA Write(VISA resource name=w892, write buffer="$2MS\u0001", error in (no error)=w891) -> ()  [unwired: 3 out]
              }
            }
            n232 = Not Equal?(x="Минуты 2", y=0) -> (x != y?=w811:bool)
            n233 = local read "положение в мин 2"() -> (w804:i32)
            n234 = Add(x="Минуты 2", y=w804) -> (x+y=w835:i32)
            n235 = Add(x="Минуты 2", y=w804) -> (x+y=w807:i32)
            n236 = Not Equal?(x="Минуты 2", y=0) -> (x != y?=w809:bool)
            n237 = Add(x=w804, y=60) -> (x+y=w830:i32)
            n238 = Subtract(x=w804, y=60) -> (x-y=w817:i32)
            n239 = Not(x=w812) -> (.not. x?=w813:bool)
            n240 = Greater Or Equal?(x=w807, y=-600) -> (x >= y?=w808:bool)
            n241 = Less Or Equal?(x=w835, y=11400) -> (x <= y?=w810:bool)
            n242 = Less Or Equal?(x=w830, y=11390) -> (x <= y?=w827:bool)
            n243 = Greater Or Equal?(x=w817, y=-590) -> (x >= y?=w818:bool)
            n244 = Compound Arithmetic op=AND(w813, w809, w808) -> (w831:bool)
            n245 = And(x=w825, y=w827) -> (x .and. y?=w826:bool)
            n246 = And(x=w824, y=w818) -> (x .and. y?=w823:bool)
            n247 = Compound Arithmetic op=AND(w812, w811, w810) -> (w833:bool)
            n248 = case shown="True" w814 {
              tunnel: [w847 w856] -> w844
              tunnel: w843 -> [w846 w855]
              tunnel: [w846 w854] -> w842
              tunnel: w841 -> [w847 w853]
              tunnel: w833 -> [_ w852]
              tunnel: w831 -> [_ w851]
              tunnel: w805 -> [_ w850]
              tunnel: w821 -> [_ w849]
              tunnel: "Минуты 2" -> [_ w848]
              frame False {
              }
              frame True {
                n249 = case shown="True" w852 {
                  tunnel: [w877 w883] -> w856
                  tunnel: w853 -> [w876 w882]
                  tunnel: w850 -> [_ w881]
                  tunnel: w849 -> [_ w880]
                  tunnel: w848 -> [_ w879]
                  frame False {
                    n250 = Add(x=0, y=w876) -> (x+y=w877:i32)
                    n251 = Wait (ms)(milliseconds to wait=u32 500) -> ()  [unwired: 1 out]
                  }
                  frame True {
                    n252 = Type Cast(type="", x=w879) -> (*(type *) &x=w886:string)
                    n253 = Add(x=w879, y=w882) -> (x+y=w883:i32)
                    n254 = String Subset(string=w886, offset (0)=1, length (rest)=3 ("length (rest)")) -> (substring=w885:string)
                    n255 = Concatenate Strings("$2MJ\u0004+" ("write buffer"), w885) -> (w889:string)
                    n256 = VISA Write(VISA resource name=w880, write buffer=w889, error in (no error)=w881) -> ()  [unwired: 3 out]
                  }
                }
                n257 = case shown="True" w851 {
                  tunnel: [w859 w865] -> w854
                  tunnel: w855 -> [w858 w864]
                  tunnel: w849 -> [_ w867]
                  tunnel: w850 -> [_ w866]
                  tunnel: w848 -> [_ w861]
                  frame False {
                    n258 = Add(x=0, y=w858) -> (x+y=w859:i32)
                    n259 = Wait (ms)(milliseconds to wait=u32 500) -> ()  [unwired: 1 out]
                  }
                  frame True {
                    n260 = Multiply(x=w861, y=-1) -> (x*y=w863:i32)
                    n261 = Type Cast(type="", x=w863) -> (*(type *) &x=w870:string)
                    n262 = Add(x=w864, y=w861) -> (x+y=w865:i32)
                    n263 = String Subset(string=w870, offset (0)=1, length (rest)=3 ("length (rest)")) -> (substring=w869:string)
                    n264 = Concatenate Strings("$2MJ\u0004-" ("write buffer"), w869) -> (w873:string)
                    n265 = VISA Write(VISA resource name=w867, write buffer=w873, error in (no error)=w866) -> ()  [unwired: 3 out]
                  }
                }
              }
            }
            n266 = case shown="True" w826 {
              tunnel: [w907 w914] -> w838
              tunnel: w840 -> [w906 w909]
              tunnel: w821 -> [_ w910]
              tunnel: w805 -> [_ w911]
              frame False {
                n267 = Add(x=0, y=w906) -> (x+y=w907:i32)
                n268 = Wait (ms)(milliseconds to wait=u32 500) -> ()  [unwired: 1 out]
              }
              frame True {
                n269 = VISA Write(VISA resource name=w910, write buffer="$2MJ\u0004+\u0000\u0000<", error in (no error)=w911) -> ()  [unwired: 3 out]
                n270 = Add(x=60, y=w909) -> (x+y=w914:i32)
              }
            }
            n271 = case shown="True" w823 {
              tunnel: [w897 w900] -> w837
              tunnel: w839 -> [w896 w899]
              tunnel: w821 -> [_ w903]
              tunnel: w805 -> [_ w902]
              frame False {
                n272 = Add(x=0, y=w896) -> (x+y=w897:i32)
                n273 = Wait (ms)(milliseconds to wait=u32 500) -> ()  [unwired: 1 out]
              }
              frame True {
                n274 = Subtract(x=w899, y=60 ("x")) -> (x-y=w900:i32)
                n275 = VISA Write(VISA resource name=w903, write buffer="$2MJ\u0004-\u0000\u0000<", error in (no error)=w902) -> ()  [unwired: 3 out]
              }
            }
            n276 = for {
              N: 1 -> [_]
              tunnel: [w845] -> w801 mode=indexing
              n277 = local read "2"() -> (w845:i32)
            }
            n278 = Index Array(array=w801, index=0) -> (element=w803:i32)
          }
          frame #2 {
            # "Нулевое положение"
            n279 = Add(x=w930, y=w931) -> (x+y=w939:i32)
            n280 = Add(x=w928, y=w929) -> (x+y=w943:i32)
            n281 = Add(x=w943, y=w939) -> (x+y=w924:i32)
            n282 = Add(x=w924, y=w915) -> (x+y=w923:i32)
            n283 = Not Equal?(x=w923, y=0 ("x")) -> (x != y?=w936:bool)
            n284 = And(x=w936, y=w938) -> (x .and. y?=w945:bool)
            n285 = case shown="True" w945 {
              tunnel: [w970 w993] -> w917
              tunnel: w928 -> [w974 w990]
              tunnel: [w974 w989] -> w946
              tunnel: [w973 w988] -> w944
              tunnel: w923 -> [w970 w982]
              tunnel: [w971 w984] -> w942
              tunnel: [w972 w981] -> w935
              tunnel: w929 -> [w973 w980]
              tunnel: w934 -> [_ w979]
              tunnel: w933 -> [_ w978]
              tunnel: w930 -> [w972 w977]
              tunnel: w931 -> [w971 w976]
              frame False {
              }
              frame True {
                n286 = Greater?(x=w982, y=0) -> (0:w983:bool)
                n287 = Multiply(x=w976, y=0) -> (x*y=w984:i32)
                n288 = Multiply(x=w980, y=0) -> (x*y=w988:i32)
                n289 = case shown="True" w983 {
                  tunnel: w982 -> [w998 w1011]
                  tunnel: [0 0] -> w993
                  tunnel: w978 -> [w995 w1008]
                  tunnel: w979 -> [w994 w1007]
                  frame False {
                    n290 = Multiply(x=w998, y=-1) -> (x*y=w996:i32)
                    n291 = Type Cast(type="", x=w996) -> (*(type *) &x=w1002:string)
                    n292 = String Subset(string=w1002, offset (0)=1, length (rest)=3 ("length (rest)")) -> (substring=w1001:string)
                    n293 = Concatenate Strings("$2MJ\u0004+" ("write buffer"), w1001) -> (w1005:string)
                    n294 = VISA Write(VISA resource name=w995, write buffer=w1005, error in (no error)=w994) -> ()  [unwired: 3 out]
                  }
                  frame True {
                    n295 = Type Cast(type="", x=w1011) -> (*(type *) &x=w1014:string)
                    n296 = String Subset(string=w1014, offset (0)=1, length (rest)=3 ("length (rest)")) -> (substring=w1013:string)
                    n297 = Concatenate Strings("$2MJ\u0004-" ("write buffer"), w1013) -> (w1009:string)
                    n298 = VISA Write(VISA resource name=w1008, write buffer=w1009, error in (no error)=w1007) -> ()  [unwired: 3 out]
                  }
                }
                n299 = Multiply(x=w977, y=0) -> (x*y=w981:i32)
                n300 = local write "2"(0 ("2")) -> ()
                n301 = Multiply(x=w990, y=0) -> (x*y=w989:i32)
              }
            }
            "положение в мин 2" <- w917
            n302 = Greater?(x=w917, y=0) -> (0:w941:bool)
            n303 = Number To Decimal String(number=w917, width (-)=i16 1) -> (decimal integer string=w926:string)
            n304 = case shown="False" w941 {
              tunnel: w917 -> [w953 w969]
              tunnel: [w957 w963] -> w921
              tunnel: [w947 w961] -> w920
              frame False {
                n305 = Multiply(x=-1, y=w953) -> (x*y=w952:i32)
                n306 = Quotient & Remainder(x=w952, y=60) -> (x-y*floor(x/y)=w956:i32, floor(x/y)=w948:i32)
                n307 = Multiply(x=-1, y=w948) -> (x*y=w947:i32)
                n308 = Number To Decimal String(number=w948) -> (decimal integer string=w954:string)  [unwired: 1 in]
                n309 = Number To Decimal String(number=w956) -> (decimal integer string=w955:string)  [unwired: 1 in]
                n310 = Concatenate Strings("-" ("string"), w954, "°" ("string"), w955, "'" ("string")) -> (w957:string)
              }
              frame True {
                n311 = Quotient & Remainder(x=w969, y=60) -> (x-y*floor(x/y)=w962:i32, floor(x/y)=w961:i32)
                n312 = Number To Decimal String(number=w962) -> (decimal integer string=w964:string)  [unwired: 1 in]
                n313 = Number To Decimal String(number=w961) -> (decimal integer string=w965:string)  [unwired: 1 in]
                n314 = Concatenate Strings(w965, "°" ("string"), w964, "'" ("string")) -> (w963:string)
              }
            }
            "положение шд 2" <- w920
            "текущее положение 2" <- w921
            n315 = Concatenate Strings(w926, "'" ("string")) -> (→"положение в минутах 2":string)
            n316 = Format Into String(w917) -> (resulting string=w918:string)  [unwired: 3 in, 1 out]
            n317 = call <vilib>:"Space Constant.vi"() -> ("String"=w916:string)
            n318 = Concatenate Strings(w916, w918) -> (→"text2":string)
          }
          frame #3 {
            # "Задача нуля"
            n319 = case shown="True" w1018 {
              tunnel: [w1030 w1042] -> w1026
              tunnel: w1025 -> [w1030 w1043]
              tunnel: w1024 -> [w1029 w1039]
              tunnel: [w1029 w1038] -> w1023
              tunnel: [w1028 w1035] -> w1022
              tunnel: [w1027 w1034] -> w1021
              tunnel: w1020 -> [w1028 w1033]
              tunnel: w1019 -> [w1027 w1032]
              frame False {
              }
              frame True {
                n320 = Multiply(x=w1039, y=0) -> (x*y=w1038:i32)
                n321 = Multiply(x=w1043, y=0) -> (x*y=w1042:i32)
                n322 = Multiply(x=w1032, y=0) -> (x*y=w1034:i32)
                n323 = Multiply(x=w1033, y=0) -> (x*y=w1035:i32)
                n324 = local write "2"(0 ("2")) -> ()
              }
            }
          }
        }
        n325 = flat-sequence {
          tunnel: w100 -> [w248]
          tunnel: w101 -> [w249]
          tunnel: [w249] -> w122
          tunnel: [w248] -> w121
          tunnel: ["Вращение по градусам +  4"] -> w120
          tunnel: ["Вращение по градусам -  4"] -> w119
          tunnel: ["Вернуться в нулевое положение 4"] -> w118
          tunnel: ["Задать текущее положение нулевым 4"] -> w117
          tunnel: ["Установка минут 4"] -> w116
          tunnel: w122 -> [w273]
          tunnel: w121 -> [w257]
          tunnel: [w296] -> w115
          tunnel: w98 -> [w293]
          tunnel: w96 -> [w295]
          tunnel: [w294] -> w114
          tunnel: w94 -> [w292]
          tunnel: w92 -> [w291]
          tunnel: w120 -> [w277]
          tunnel: w119 -> [w276]
          tunnel: [w290] -> w113
          tunnel: [w289] -> w112
          tunnel: [w274] -> w111
          tunnel: w118 -> [w274]
          tunnel: [w257] -> w110
          tunnel: [w273] -> w109
          tunnel: [w272] -> w108
          tunnel: w117 -> [w272]
          tunnel: w116 -> [w266]
          tunnel: [w255] -> w107
          tunnel: w115 -> [w380]
          tunnel: w114 -> [w381]
          tunnel: [w398] -> w106
          tunnel: [w396] -> w105
          tunnel: w113 -> [w382]
          tunnel: w112 -> [w383]
          tunnel: [w387] -> w104
          tunnel: [w394] -> w103
          tunnel: w111 -> [w390]
          tunnel: w110 -> [w386]
          tunnel: w109 -> [w385]
          tunnel: w108 -> [w384]
          tunnel: [w384] -> w102
          tunnel: w107 -> [w370]
          tunnel: [w478] -> w97
          tunnel: [w475] -> w95
          tunnel: w106 -> [w477]
          tunnel: w105 -> [w476]
          tunnel: [w474] -> w93
          tunnel: [w473] -> w91
          tunnel: w104 -> [w472]
          tunnel: w103 -> [w471]
          tunnel: w102 -> [w470]
          frame #0 {
            n326 = Wait Until Next ms Multiple(millisecond multiple=u32 300) -> ()  [unwired: 1 out]
          }
          frame #1 {
            # "Остановка двигателя"
            n327 = Greater?(x="Минуты 4", y=0) -> (0:w264:bool)
            n328 = case shown="True" "Stop двигатель 4" {
              tunnel: w273 -> [_ w344]
              tunnel: w257 -> [_ w343]
              frame False {
              }
              frame True {
                n329 = Wait (ms)(milliseconds to wait=u32 500) -> ()  [unwired: 1 out]
                n330 = VISA Write(VISA resource name=w344, write buffer="$4MS\u0001", error in (no error)=w343) -> ()  [unwired: 3 out]
              }
            }
            n331 = Not Equal?(x="Минуты 4", y=0) -> (x != y?=w263:bool)
            n332 = local read "положение в мин 4"() -> (w256:i32)
            n333 = Add(x="Минуты 4", y=w256) -> (x+y=w287:i32)
            n334 = Add(x="Минуты 4", y=w256) -> (x+y=w259:i32)
            n335 = Not Equal?(x="Минуты 4", y=0) -> (x != y?=w261:bool)
            n336 = Add(x=w256, y=60) -> (x+y=w282:i32)
            n337 = Subtract(x=w256, y=60) -> (x-y=w269:i32)
            n338 = Not(x=w264) -> (.not. x?=w265:bool)
            n339 = Greater Or Equal?(x=w259, y=-600) -> (x >= y?=w260:bool)
            n340 = Less Or Equal?(x=w287, y=11400) -> (x <= y?=w262:bool)
            n341 = Less Or Equal?(x=w282, y=11390) -> (x <= y?=w279:bool)
            n342 = Greater Or Equal?(x=w269, y=-590) -> (x >= y?=w270:bool)
            n343 = Compound Arithmetic op=AND(w265, w261, w260) -> (w283:bool)
            n344 = And(x=w277, y=w279) -> (x .and. y?=w278:bool)
            n345 = And(x=w276, y=w270) -> (x .and. y?=w275:bool)
            n346 = Compound Arithmetic op=AND(w264, w263, w262) -> (w285:bool)
            n347 = case shown="True" w266 {
              tunnel: [w299 w308] -> w296
              tunnel: w295 -> [w298 w307]
              tunnel: [w298 w306] -> w294
              tunnel: w293 -> [w299 w305]
              tunnel: w285 -> [_ w304]
              tunnel: w283 -> [_ w303]
              tunnel: w257 -> [_ w302]
              tunnel: w273 -> [_ w301]
              tunnel: "Минуты 4" -> [_ w300]
              frame False {
              }
              frame True {
                n348 = case shown="True" w304 {
                  tunnel: [w329 w335] -> w308
                  tunnel: w305 -> [w328 w334]
                  tunnel: w302 -> [_ w333]
                  tunnel: w301 -> [_ w332]
                  tunnel: w300 -> [_ w331]
                  frame False {
                    n349 = Add(x=0, y=w328) -> (x+y=w329:i32)
                    n350 = Wait (ms)(milliseconds to wait=u32 500) -> ()  [unwired: 1 out]
                  }
                  frame True {
                    n351 = Type Cast(type="", x=w331) -> (*(type *) &x=w338:string)
                    n352 = Add(x=w331, y=w334) -> (x+y=w335:i32)
                    n353 = String Subset(string=w338, offset (0)=1, length (rest)=3 ("length (rest)")) -> (substring=w337:string)
                    n354 = Concatenate Strings("$4MJ\u0004+" ("write buffer"), w337) -> (w341:string)
                    n355 = VISA Write(VISA resource name=w332, write buffer=w341, error in (no error)=w333) -> ()  [unwired: 3 out]
                  }
                }
                n356 = case shown="True" w303 {
                  tunnel: [w311 w317] -> w306
                  tunnel: w307 -> [w310 w316]
                  tunnel: w301 -> [_ w319]
                  tunnel: w302 -> [_ w318]
                  tunnel: w300 -> [_ w313]
                  frame False {
                    n357 = Add(x=0, y=w310) -> (x+y=w311:i32)
                    n358 = Wait (ms)(milliseconds to wait=u32 500) -> ()  [unwired: 1 out]
                  }
                  frame True {
                    n359 = Multiply(x=w313, y=-1) -> (x*y=w315:i32)
                    n360 = Type Cast(type="", x=w315) -> (*(type *) &x=w322:string)
                    n361 = Add(x=w316, y=w313) -> (x+y=w317:i32)
                    n362 = String Subset(string=w322, offset (0)=1, length (rest)=3 ("length (rest)")) -> (substring=w321:string)
                    n363 = Concatenate Strings("$4MJ\u0004-" ("write buffer"), w321) -> (w325:string)
                    n364 = VISA Write(VISA resource name=w319, write buffer=w325, error in (no error)=w318) -> ()  [unwired: 3 out]
                  }
                }
              }
            }
            n365 = case shown="True" w278 {
              tunnel: [w359 w366] -> w290
              tunnel: w292 -> [w358 w361]
              tunnel: w273 -> [_ w362]
              tunnel: w257 -> [_ w363]
              frame False {
                n366 = Add(x=0, y=w358) -> (x+y=w359:i32)
                n367 = Wait (ms)(milliseconds to wait=u32 500) -> ()  [unwired: 1 out]
              }
              frame True {
                n368 = VISA Write(VISA resource name=w362, write buffer="$4MJ\u0004+\u0000\u0000<", error in (no error)=w363) -> ()  [unwired: 3 out]
                n369 = Add(x=60, y=w361) -> (x+y=w366:i32)
              }
            }
            n370 = case shown="True" w275 {
              tunnel: [w349 w352] -> w289
              tunnel: w291 -> [w348 w351]
              tunnel: w273 -> [_ w355]
              tunnel: w257 -> [_ w354]
              frame False {
                n371 = Add(x=0, y=w348) -> (x+y=w349:i32)
                n372 = Wait (ms)(milliseconds to wait=u32 500) -> ()  [unwired: 1 out]
              }
              frame True {
                n373 = Subtract(x=w351, y=60 ("x")) -> (x-y=w352:i32)
                n374 = VISA Write(VISA resource name=w355, write buffer="$4MJ\u0004-\u0000\u0000<", error in (no error)=w354) -> ()  [unwired: 3 out]
              }
            }
            n375 = for {
              N: 1 -> [_]
              tunnel: [w297] -> w253 mode=indexing
              n376 = local read "4"() -> (w297:i32)
            }
            n377 = Index Array(array=w253, index=0) -> (element=w255:i32)
          }
          frame #2 {
            # "Нулевое положение"
            n378 = Add(x=w382, y=w383) -> (x+y=w391:i32)
            n379 = Add(x=w380, y=w381) -> (x+y=w395:i32)
            n380 = Add(x=w395, y=w391) -> (x+y=w376:i32)
            n381 = Add(x=w376, y=w370) -> (x+y=w375:i32)
            n382 = Not Equal?(x=w375, y=0 ("x")) -> (x != y?=w388:bool)
            n383 = And(x=w388, y=w390) -> (x .and. y?=w397:bool)
            n384 = case shown="True" w397 {
              tunnel: [w422 w445] -> w372
              tunnel: w380 -> [w426 w442]
              tunnel: [w426 w441] -> w398
              tunnel: [w425 w440] -> w396
              tunnel: w375 -> [w422 w434]
              tunnel: [w423 w436] -> w394
              tunnel: [w424 w433] -> w387
              tunnel: w381 -> [w425 w432]
              tunnel: w386 -> [_ w431]
              tunnel: w385 -> [_ w430]
              tunnel: w382 -> [w424 w429]
              tunnel: w383 -> [w423 w428]
              frame False {
              }
              frame True {
                n385 = Greater?(x=w434, y=0) -> (0:w435:bool)
                n386 = Multiply(x=w428, y=0) -> (x*y=w436:i32)
                n387 = Multiply(x=w432, y=0) -> (x*y=w440:i32)
                n388 = case shown="True" w435 {
                  tunnel: w434 -> [w450 w463]
                  tunnel: [0 0] -> w445
                  tunnel: w430 -> [w447 w460]
                  tunnel: w431 -> [w446 w459]
                  frame False {
                    n389 = Multiply(x=w450, y=-1) -> (x*y=w448:i32)
                    n390 = Type Cast(type="", x=w448) -> (*(type *) &x=w454:string)
                    n391 = String Subset(string=w454, offset (0)=1, length (rest)=3 ("length (rest)")) -> (substring=w453:string)
                    n392 = Concatenate Strings("$4MJ\u0004+" ("write buffer"), w453) -> (w457:string)
                    n393 = VISA Write(VISA resource name=w447, write buffer=w457, error in (no error)=w446) -> ()  [unwired: 3 out]
                  }
                  frame True {
                    n394 = Type Cast(type="", x=w463) -> (*(type *) &x=w466:string)
                    n395 = String Subset(string=w466, offset (0)=1, length (rest)=3 ("length (rest)")) -> (substring=w465:string)
                    n396 = Concatenate Strings("$4MJ\u0004-" ("write buffer"), w465) -> (w461:string)
                    n397 = VISA Write(VISA resource name=w460, write buffer=w461, error in (no error)=w459) -> ()  [unwired: 3 out]
                  }
                }
                n398 = Multiply(x=w429, y=0) -> (x*y=w433:i32)
                n399 = Multiply(x=w442, y=0) -> (x*y=w441:i32)
                n400 = local write "4"(0 ("4")) -> ()
              }
            }
            "положение в мин 4" <- w372
            n401 = Greater?(x=w372, y=0) -> (0:w393:bool)
            n402 = Number To Decimal String(number=w372, width (-)=i16 1) -> (decimal integer string=w378:string)
            n403 = case shown="False" w393 {
              tunnel: w372 -> [w405 w421]
              tunnel: [w409 w415] -> w368
              tunnel: [w399 w413] -> w369
              frame False {
                n404 = Multiply(x=-1, y=w405) -> (x*y=w404:i32)
                n405 = Quotient & Remainder(x=w404, y=60) -> (x-y*floor(x/y)=w408:i32, floor(x/y)=w400:i32)
                n406 = Multiply(x=-1, y=w400) -> (x*y=w399:i32)
                n407 = Number To Decimal String(number=w400) -> (decimal integer string=w406:string)  [unwired: 1 in]
                n408 = Number To Decimal String(number=w408) -> (decimal integer string=w407:string)  [unwired: 1 in]
                n409 = Concatenate Strings("-" ("string"), w406, "°" ("string"), w407, "'" ("string")) -> (w409:string)
              }
              frame True {
                n410 = Quotient & Remainder(x=w421, y=60) -> (x-y*floor(x/y)=w414:i32, floor(x/y)=w413:i32)
                n411 = Number To Decimal String(number=w414) -> (decimal integer string=w416:string)  [unwired: 1 in]
                n412 = Number To Decimal String(number=w413) -> (decimal integer string=w417:string)  [unwired: 1 in]
                n413 = Concatenate Strings(w417, "°" ("string"), w416, "'" ("string")) -> (w415:string)
              }
            }
            "положение шд 4" <- w369
            "текущее положение 4" <- w368
            n414 = Concatenate Strings(w378, "'" ("string")) -> (→"положение в минутах 4":string)
            n415 = Format Into String(w372) -> (resulting string=w373:string)  [unwired: 3 in, 1 out]
            n416 = call <vilib>:"Space Constant.vi"() -> ("String"=w371:string)
            n417 = Concatenate Strings(w371, w373) -> (→"text4":string)
          }
          frame #3 {
            # "Задача нуля"
            n418 = case shown="True" w470 {
              tunnel: [w482 w494] -> w478
              tunnel: w477 -> [w482 w495]
              tunnel: w476 -> [w481 w491]
              tunnel: [w481 w490] -> w475
              tunnel: [w480 w487] -> w474
              tunnel: [w479 w486] -> w473
              tunnel: w472 -> [w480 w485]
              tunnel: w471 -> [w479 w484]
              frame False {
              }
              frame True {
                n419 = Multiply(x=w491, y=0) -> (x*y=w490:i32)
                n420 = Multiply(x=w495, y=0) -> (x*y=w494:i32)
                n421 = local write "4"(0 ("4")) -> ()
                n422 = Multiply(x=w484, y=0) -> (x*y=w486:i32)
                n423 = Multiply(x=w485, y=0) -> (x*y=w487:i32)
              }
            }
          }
        }
        n424 = case shown="True" "Блокировать трубку №2" {
          frame False {
            n425 = property on="Stop двигатель 2" class="Bool"("DisabledEnum"=T3."Enabled" ("Disabled")) -> ()  [unwired: 2 in, 2 out]
            n426 = property on="Вернуться в нулевое положение 2" class="Bool"("DisabledEnum"=T3."Enabled" ("Disabled")) -> ()  [unwired: 2 in, 2 out]
            n427 = property on="Вращение по градусам +  2" class="Bool"("DisabledEnum"=T3."Enabled" ("Disabled")) -> ()  [unwired: 2 in, 2 out]
            n428 = property on="текущее положение 2" class="Str"("DisabledEnum"=T3."Enabled" ("Disabled")) -> ()  [unwired: 2 in, 2 out]
            n429 = property on="Установка минут 2" class="Bool"("DisabledEnum"=T3."Enabled" ("Disabled")) -> ()  [unwired: 2 in, 2 out]
            n430 = property on="Вращение по градусам -  2" class="Bool"("DisabledEnum"=T3."Enabled" ("Disabled")) -> ()  [unwired: 2 in, 2 out]
            n431 = property on="Задать текущее положение нулевым 2" class="Bool"("DisabledEnum"=T3."Enabled" ("Disabled")) -> ()  [unwired: 2 in, 2 out]
            n432 = property on="Минуты 2" class="DigNum (strict)"("DisabledEnum"=T3."Enabled" ("Disabled")) -> ()  [unwired: 2 in, 2 out]
            n433 = property on="положение шд 2" class="Knob (strict)"("DisabledEnum"=T3."Enabled" ("Disabled")) -> ()  [unwired: 2 in, 2 out]
            n434 = property on="положение в минутах 2" class="Str"("DisabledEnum"=T3."Enabled" ("Disabled")) -> ()  [unwired: 2 in, 2 out]
          }
          frame True {
            n435 = property on="Вернуться в нулевое положение 2" class="Bool"("DisabledEnum"=T3."Disabled and Grayed Out" ("Disabled")) -> ()  [unwired: 2 in, 2 out]
            n436 = property on="положение шд 2" class="Knob (strict)"("DisabledEnum"=T3."Disabled and Grayed Out" ("Disabled")) -> ()  [unwired: 2 in, 2 out]
            n437 = property on="текущее положение 2" class="Str"("DisabledEnum"=T3."Disabled and Grayed Out" ("Disabled")) -> ()  [unwired: 2 in, 2 out]
            n438 = property on="Stop двигатель 2" class="Bool"("DisabledEnum"=T3."Disabled and Grayed Out" ("Disabled")) -> ()  [unwired: 2 in, 2 out]
            n439 = property on="Вращение по градусам +  2" class="Bool"("DisabledEnum"=T3."Disabled and Grayed Out" ("Disabled")) -> ()  [unwired: 2 in, 2 out]
            n440 = property on="Вращение по градусам -  2" class="Bool"("DisabledEnum"=T3."Disabled and Grayed Out" ("Disabled")) -> ()  [unwired: 2 in, 2 out]
            n441 = property on="Задать текущее положение нулевым 2" class="Bool"("DisabledEnum"=T3."Disabled and Grayed Out" ("Disabled")) -> ()  [unwired: 2 in, 2 out]
            n442 = property on="Минуты 2" class="DigNum (strict)"("DisabledEnum"=T3."Disabled and Grayed Out" ("Disabled")) -> ()  [unwired: 2 in, 2 out]
            n443 = property on="Установка минут 2" class="Bool"("DisabledEnum"=T3."Disabled and Grayed Out" ("Disabled")) -> ()  [unwired: 2 in, 2 out]
            n444 = property on="положение в минутах 2" class="Str"("DisabledEnum"=T3."Disabled and Grayed Out" ("Disabled")) -> ()  [unwired: 2 in, 2 out]
          }
        }
        n445 = case shown="False" "Блокировать стол №3" {
          frame False {
            n446 = property on="Stop двигатель 3" class="Bool"("DisabledEnum"=T3."Enabled" ("Disabled")) -> ()  [unwired: 2 in, 2 out]
            n447 = property on="Вернуться в нулевое положение 3" class="Bool"("DisabledEnum"=T3."Enabled" ("Disabled")) -> ()  [unwired: 2 in, 2 out]
            n448 = property on="Вращение по градусам +  3" class="Bool"("DisabledEnum"=T3."Enabled" ("Disabled")) -> ()  [unwired: 2 in, 2 out]
            n449 = property on="текущее положение 3" class="Str"("DisabledEnum"=T3."Enabled" ("Disabled")) -> ()  [unwired: 2 in, 2 out]
            n450 = property on="Установка минут 3" class="Bool"("DisabledEnum"=T3."Enabled" ("Disabled")) -> ()  [unwired: 2 in, 2 out]
            n451 = property on="Вращение по градусам -  3" class="Bool"("DisabledEnum"=T3."Enabled" ("Disabled")) -> ()  [unwired: 2 in, 2 out]
            n452 = property on="Задать текущее положение нулевым 3" class="Bool"("DisabledEnum"=T3."Enabled" ("Disabled")) -> ()  [unwired: 2 in, 2 out]
            n453 = property on="Минуты 3" class="DigNum (strict)"("DisabledEnum"=T3."Enabled" ("Disabled")) -> ()  [unwired: 2 in, 2 out]
            n454 = property on="положение шд 3" class="Knob (strict)"("DisabledEnum"=T3."Enabled" ("Disabled")) -> ()  [unwired: 2 in, 2 out]
            n455 = property on="положение в минутах 3" class="Str"("DisabledEnum"=T3."Enabled" ("Disabled")) -> ()  [unwired: 2 in, 2 out]
          }
          frame True {
            n456 = property on="Вернуться в нулевое положение 3" class="Bool"("DisabledEnum"=T3."Disabled and Grayed Out" ("Disabled")) -> ()  [unwired: 2 in, 2 out]
            n457 = property on="положение шд 3" class="Knob (strict)"("DisabledEnum"=T3."Disabled and Grayed Out" ("Disabled")) -> ()  [unwired: 2 in, 2 out]
            n458 = property on="текущее положение 3" class="Str"("DisabledEnum"=T3."Disabled and Grayed Out" ("Disabled")) -> ()  [unwired: 2 in, 2 out]
            n459 = property on="Stop двигатель 3" class="Bool"("DisabledEnum"=T3."Disabled and Grayed Out" ("Disabled")) -> ()  [unwired: 2 in, 2 out]
            n460 = property on="Вращение по градусам +  3" class="Bool"("DisabledEnum"=T3."Disabled and Grayed Out" ("Disabled")) -> ()  [unwired: 2 in, 2 out]
            n461 = property on="Вращение по градусам -  3" class="Bool"("DisabledEnum"=T3."Disabled and Grayed Out" ("Disabled")) -> ()  [unwired: 2 in, 2 out]
            n462 = property on="Задать текущее положение нулевым 3" class="Bool"("DisabledEnum"=T3."Disabled and Grayed Out" ("Disabled")) -> ()  [unwired: 2 in, 2 out]
            n463 = property on="Минуты 3" class="DigNum (strict)"("DisabledEnum"=T3."Disabled and Grayed Out" ("Disabled")) -> ()  [unwired: 2 in, 2 out]
            n464 = property on="Установка минут 3" class="Bool"("DisabledEnum"=T3."Disabled and Grayed Out" ("Disabled")) -> ()  [unwired: 2 in, 2 out]
            n465 = property on="положение в минутах 3" class="Str"("DisabledEnum"=T3."Disabled and Grayed Out" ("Disabled")) -> ()  [unwired: 2 in, 2 out]
          }
        }
        n466 = case shown="False" "Блокировать зеркало №1" {
          frame False {
            n467 = property on="Stop двигатель" class="Bool"("DisabledEnum"=T3."Enabled" ("Disabled")) -> ()  [unwired: 2 in, 2 out]
            n468 = property on="Вернуться в нулевое положение" class="Bool"("DisabledEnum"=T3."Enabled" ("Disabled")) -> ()  [unwired: 2 in, 2 out]
            n469 = property on="Вращение по градусам +" class="Bool"("DisabledEnum"=T3."Enabled" ("Disabled")) -> ()  [unwired: 2 in, 2 out]
            n470 = property on="текущее положение" class="Str"("DisabledEnum"=T3."Enabled" ("Disabled")) -> ()  [unwired: 2 in, 2 out]
            n471 = property on="Установка минут" class="Bool"("DisabledEnum"=T3."Enabled" ("Disabled")) -> ()  [unwired: 2 in, 2 out]
            n472 = property on="Вращение по градусам -" class="Bool"("DisabledEnum"=T3."Enabled" ("Disabled")) -> ()  [unwired: 2 in, 2 out]
            n473 = property on="Задать текущее положение нулевым" class="Bool"("DisabledEnum"=T3."Enabled" ("Disabled")) -> ()  [unwired: 2 in, 2 out]
            n474 = property on="Минуты" class="DigNum (strict)"("DisabledEnum"=T3."Enabled" ("Disabled")) -> ()  [unwired: 2 in, 2 out]
            n475 = property on="положение шд" class="Knob (strict)"("DisabledEnum"=T3."Enabled" ("Disabled")) -> ()  [unwired: 2 in, 2 out]
            n476 = property on="положение в минутах 1" class="Str"("DisabledEnum"=T3."Enabled" ("Disabled")) -> ()  [unwired: 2 in, 2 out]
          }
          frame True {
            n477 = property on="Вернуться в нулевое положение" class="Bool"("DisabledEnum"=T3."Disabled and Grayed Out" ("Disabled")) -> ()  [unwired: 2 in, 2 out]
            n478 = property on="положение шд" class="Knob (strict)"("DisabledEnum"=T3."Disabled and Grayed Out" ("Disabled")) -> ()  [unwired: 2 in, 2 out]
            n479 = property on="текущее положение" class="Str"("DisabledEnum"=T3."Disabled and Grayed Out" ("Disabled")) -> ()  [unwired: 2 in, 2 out]
            n480 = property on="Stop двигатель" class="Bool"("DisabledEnum"=T3."Disabled and Grayed Out" ("Disabled")) -> ()  [unwired: 2 in, 2 out]
            n481 = property on="Вращение по градусам +" class="Bool"("DisabledEnum"=T3."Disabled and Grayed Out" ("Disabled")) -> ()  [unwired: 2 in, 2 out]
            n482 = property on="Вращение по градусам -" class="Bool"("DisabledEnum"=T3."Disabled and Grayed Out" ("Disabled")) -> ()  [unwired: 2 in, 2 out]
            n483 = property on="Задать текущее положение нулевым" class="Bool"("DisabledEnum"=T3."Disabled and Grayed Out" ("Disabled")) -> ()  [unwired: 2 in, 2 out]
            n484 = property on="Минуты" class="DigNum (strict)"("DisabledEnum"=T3."Disabled and Grayed Out" ("Disabled")) -> ()  [unwired: 2 in, 2 out]
            n485 = property on="Установка минут" class="Bool"("DisabledEnum"=T3."Disabled and Grayed Out" ("Disabled")) -> ()  [unwired: 2 in, 2 out]
            n486 = property on="положение в минутах 1" class="Str"("DisabledEnum"=T3."Disabled and Grayed Out" ("Disabled")) -> ()  [unwired: 2 in, 2 out]
          }
        }
        n487 = case shown="False" "Блокировать стол №3 2" {
          frame False {
            n488 = property on="Stop двигатель 4" class="Bool"("DisabledEnum"=T3."Enabled" ("Disabled")) -> ()  [unwired: 2 in, 2 out]
            n489 = property on="Вернуться в нулевое положение 4" class="Bool"("DisabledEnum"=T3."Enabled" ("Disabled")) -> ()  [unwired: 2 in, 2 out]
            n490 = property on="Вращение по градусам +  4" class="Bool"("DisabledEnum"=T3."Enabled" ("Disabled")) -> ()  [unwired: 2 in, 2 out]
            n491 = property on="текущее положение 4" class="Str"("DisabledEnum"=T3."Enabled" ("Disabled")) -> ()  [unwired: 2 in, 2 out]
            n492 = property on="Установка минут 4" class="Bool"("DisabledEnum"=T3."Enabled" ("Disabled")) -> ()  [unwired: 2 in, 2 out]
            n493 = property on="Вращение по градусам -  4" class="Bool"("DisabledEnum"=T3."Enabled" ("Disabled")) -> ()  [unwired: 2 in, 2 out]
            n494 = property on="Задать текущее положение нулевым 4" class="Bool"("DisabledEnum"=T3."Enabled" ("Disabled")) -> ()  [unwired: 2 in, 2 out]
            n495 = property on="Минуты 4" class="DigNum (strict)"("DisabledEnum"=T3."Enabled" ("Disabled")) -> ()  [unwired: 2 in, 2 out]
            n496 = property on="положение шд 4" class="Knob (strict)"("DisabledEnum"=T3."Enabled" ("Disabled")) -> ()  [unwired: 2 in, 2 out]
            n497 = property on="положение в минутах 4" class="Str"("DisabledEnum"=T3."Enabled" ("Disabled")) -> ()  [unwired: 2 in, 2 out]
          }
          frame True {
            n498 = property on="Вернуться в нулевое положение 4" class="Bool"("DisabledEnum"=T3."Disabled and Grayed Out" ("Disabled")) -> ()  [unwired: 2 in, 2 out]
            n499 = property on="положение шд 4" class="Knob (strict)"("DisabledEnum"=T3."Disabled and Grayed Out" ("Disabled")) -> ()  [unwired: 2 in, 2 out]
            n500 = property on="текущее положение 4" class="Str"("DisabledEnum"=T3."Disabled and Grayed Out" ("Disabled")) -> ()  [unwired: 2 in, 2 out]
            n501 = property on="Stop двигатель 4" class="Bool"("DisabledEnum"=T3."Disabled and Grayed Out" ("Disabled")) -> ()  [unwired: 2 in, 2 out]
            n502 = property on="Вращение по градусам +  4" class="Bool"("DisabledEnum"=T3."Disabled and Grayed Out" ("Disabled")) -> ()  [unwired: 2 in, 2 out]
            n503 = property on="Вращение по градусам -  4" class="Bool"("DisabledEnum"=T3."Disabled and Grayed Out" ("Disabled")) -> ()  [unwired: 2 in, 2 out]
            n504 = property on="Задать текущее положение нулевым 4" class="Bool"("DisabledEnum"=T3."Disabled and Grayed Out" ("Disabled")) -> ()  [unwired: 2 in, 2 out]
            n505 = property on="Минуты 4" class="DigNum (strict)"("DisabledEnum"=T3."Disabled and Grayed Out" ("Disabled")) -> ()  [unwired: 2 in, 2 out]
            n506 = property on="Установка минут 4" class="Bool"("DisabledEnum"=T3."Disabled and Grayed Out" ("Disabled")) -> ()  [unwired: 2 in, 2 out]
            n507 = property on="положение в минутах 4" class="Str"("DisabledEnum"=T3."Disabled and Grayed Out" ("Disabled")) -> ()  [unwired: 2 in, 2 out]
          }
        }
      }
      n508 = Close File(refnum=w86) -> ()  [unwired: 1 in, 2 out]
    }
  }
